vi "Send Message Normal.vi"(4 "Source (\"\")":string, 6 "Timeout (25000)":u32=25000, 8 "error in (no error)":errorcluster, 10 "Send Message (\"\")":string, 11 "VISA resource name":refnum<visa-resource-name>) -> (0 "error out":errorcluster, 1 "Read Buffer":string, 3 "VISA resource name out":refnum<visa-resource-name>)   [LabVIEW 2020, in "Yokogawa GX Series.lvlib"]
doc: "This VI sends the message. Then it returns the response."
uses:
  <instrlib>/Yokogawa GX Series/Yokogawa GX Series.lvlib
panel:
  # "msec"
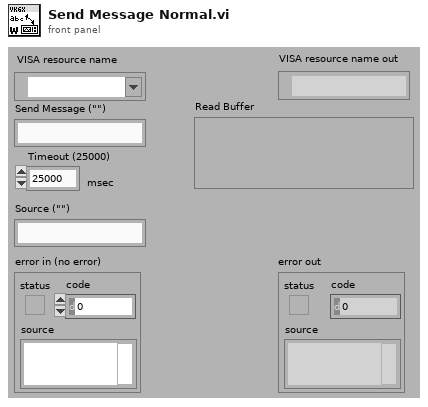
[diagram p1: front panel]
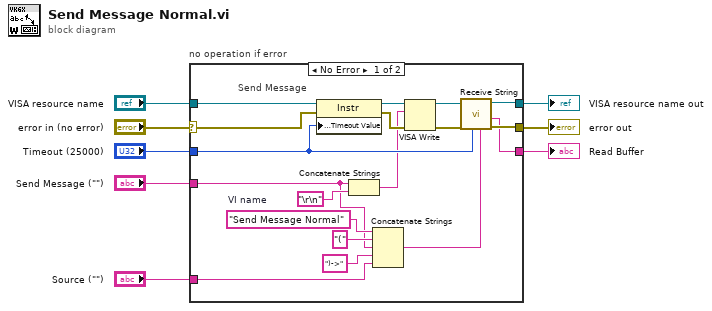
[diagram p0: block diagram]
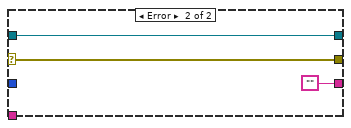
[diagram p2: hidden frame]
diagram:
  n1 = case "no operation if error" shown="No Error" "error in (no error)" {
    selector: "error in (no error)" -> [w17 w28]
    tunnel: "VISA resource name" -> [w25 w29]
    tunnel: "Send Message (\"\")" -> [w9 _]
    tunnel: [w20 w29] -> w5
    tunnel: [w19 w28] -> w8
    tunnel: "Timeout (25000)" -> [w23 _]
    tunnel: [w18 ""] -> w6
    tunnel: "Source (\"\")" -> [w12 _]
    frame No Error {
      w16 = "Send Message Normal"  # VI name
      # "Send Message"
      n2 = property class="Instr"(reference=w25, error in=w17, "General Settings:Timeout Value"=w23) -> (reference out=w24:refnum<visa-resource-name>, error out=w26:errorcluster)
      n3 = Concatenate Strings(w9, "\r\n") -> (w11:string)
      n4 = Concatenate Strings(w16, "(", w9, ")->", w12) -> (w10:string)
      n5 = VISA Write(VISA resource name=w24, write buffer=w11, error in (no error)=w26) -> (VISA resource name out=w21:refnum<visa-resource-name>, error out=w22:errorcluster)  [unwired: 1 out]
      n6 = call <instrlib>:"Receive String.vi"("Source (\"\")"=w10, "Timeout (25000)"=w23, "error in (no error)"=w22, "VISA resource name"=w21) -> ("error out"=w19:errorcluster, "Read Buffer"=w18:string, "VISA resource name out"=w20:refnum<visa-resource-name>)  [unwired: 5 out]
    }
    frame Error {
    }
  }
  "error out" <- w8
  "VISA resource name out" <- w5
  "Read Buffer" <- w6
